vi "Power Supply Global.vi"(0 "Closed Loop":bool, 2 "PS Global Mode":T1=enum."Read", 5 "PS Cmd":dbl min=0.0 max=20.0 format="%#.2f", 7 "PS Voltage":dbl, 9 "FreezePID":bool, 11 "VoltCtrlRef":string) -> (4 "Closed Loop OUT":bool, 6 "PS Cmd OUT":dbl, 8 "PS Voltage OUT":dbl, 10 "FreezePID OUT":bool, 15 "VoltCtrlRef OUT":string)   [LabVIEW 2019]
uses:
  Controls/Power Supply Global Mode.ctl
panel:
  in  "Power Supply Cmd (V):":dbl min=0.0 max=20.0 format="%#.2f"
  in  "Closed Loop Voltage":bool
  out "FreezePID":bool
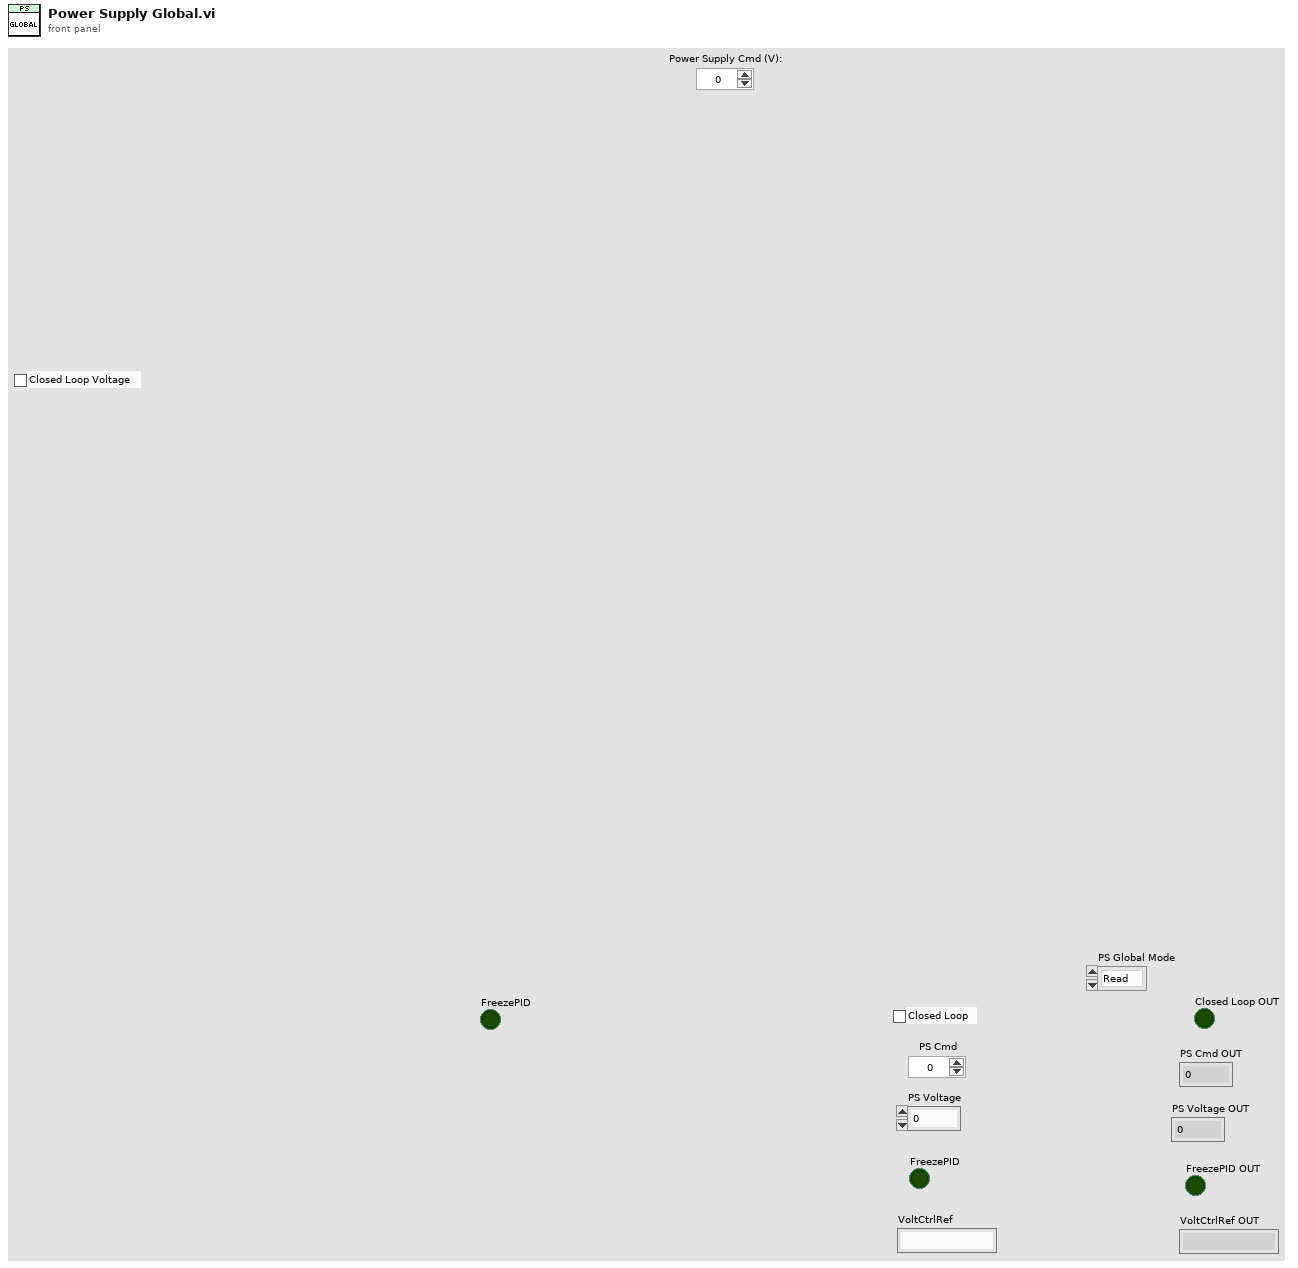
[diagram p1: front panel]
types:
  T1 = typedef "Power Supply Global Mode.ctl" = enum16{"Write Setpoint", "Write FreezePID", "Read"}
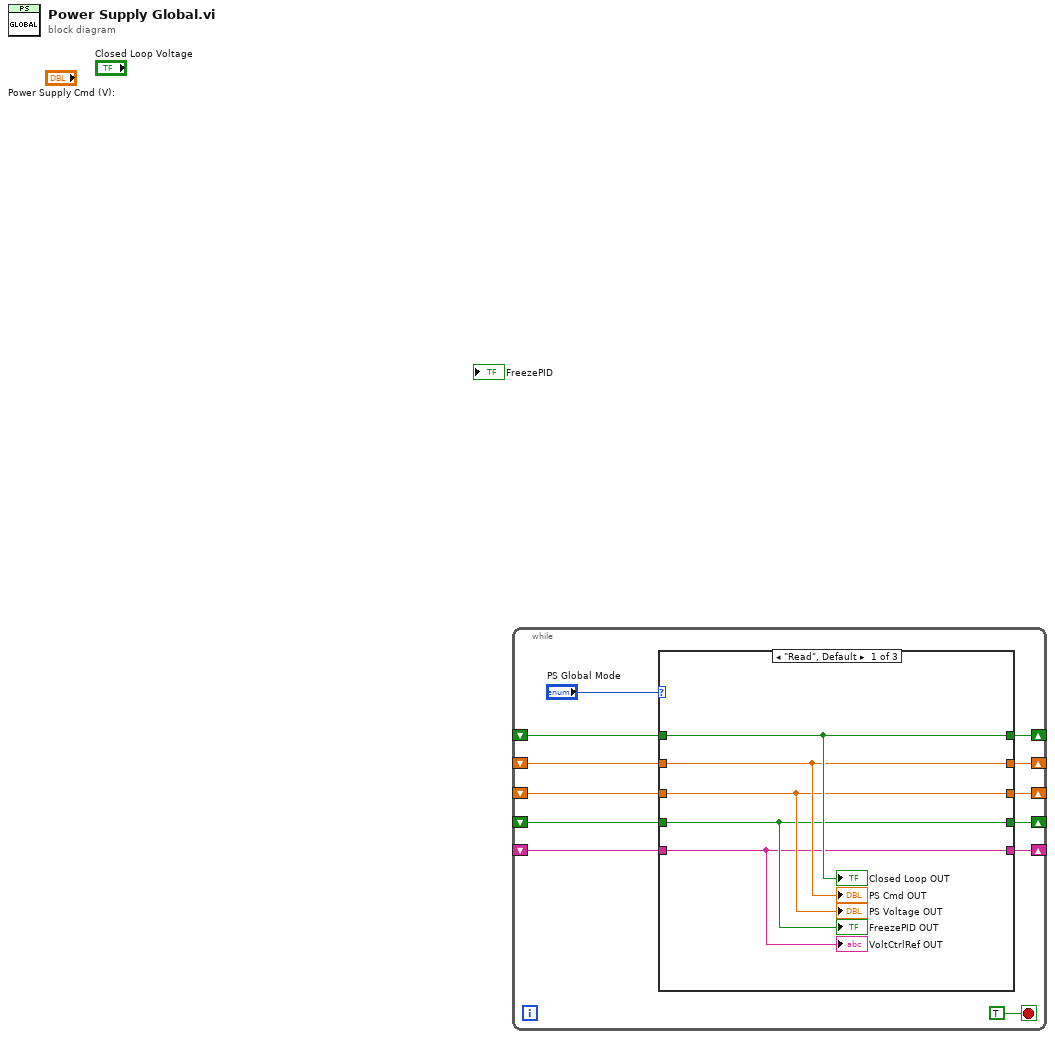
[diagram p0: block diagram]
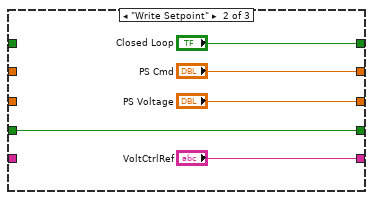
[diagram p2: hidden frame]
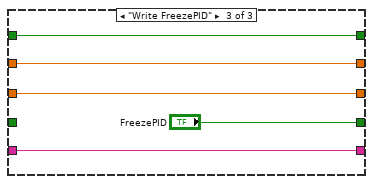
[diagram p3: hidden frame]
diagram:
  n1 = while {
    shift-right: [w11] -> _
    shift-left: _ -> [w7]
    shift-right: [w10] -> _
    shift-left: _ -> [w6]
    shift-right: [w9] -> _
    shift-left: _ -> [w5]
    shift-right: [w8] -> _
    shift-left: _ -> [w4]
    shift-right: [w2] -> _
    shift-left: _ -> [w1]
    stop <- TRUE stop-if-true
    n2 = case shown="\"Read\", Default" "PS Global Mode" {
      tunnel: [w17 "Closed Loop" w27] -> w11
      tunnel: [w16 "PS Cmd" w26] -> w10
      tunnel: [w15 "PS Voltage" w25] -> w9
      tunnel: [w14 w19 "FreezePID"] -> w8
      tunnel: w7 -> [w17 _ w27]
      tunnel: w6 -> [w16 _ w26]
      tunnel: w5 -> [w15 _ w25]
      tunnel: w4 -> [w14 w19 _]
      tunnel: [w13 "VoltCtrlRef" w23] -> w2
      tunnel: w1 -> [w13 _ w23]
      frame "Read", Default {
        "Closed Loop OUT" <- w17
        "PS Cmd OUT" <- w16
        "PS Voltage OUT" <- w15
        "FreezePID OUT" <- w14
        "VoltCtrlRef OUT" <- w13
      }
      frame "Write Setpoint" {
      }
      frame "Write FreezePID" {
      }
    }
  }
